vi "Write DataDVR.vi"(8 "error in (no error)":errorcluster, 10 "DataDVR":refnum<data-value>, 11 "gController in":refnum<class "gController.lvclass">) -> (0 "error out":errorcluster, 3 "gController out":refnum<class "gController.lvclass">)   [LabVIEW 2016, in "Controller.lvlib" / "gController.lvclass"]
uses:
  gController.lvclass
  Data/gData/gData.lvclass
  gController.lvclass/gController.ctl
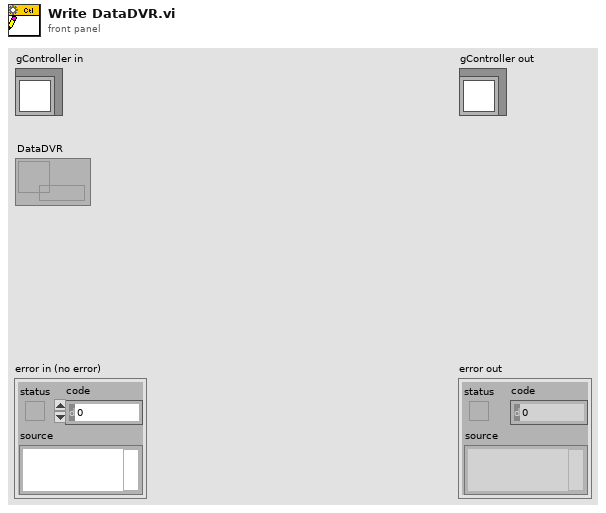
[diagram p1: front panel]
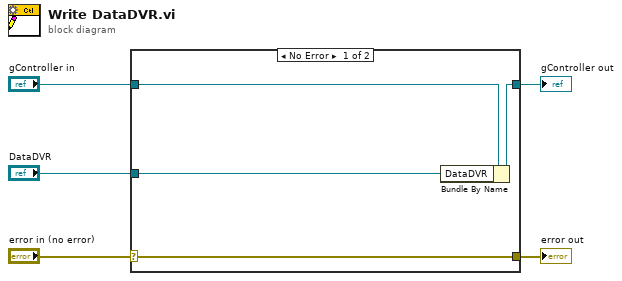
[diagram p0: block diagram]
diagram:
  n1 = case shown="No Error" "error in (no error)" {
    selector: "error in (no error)" -> [w9 w10]
    tunnel: [w9 w10] -> w4
    tunnel: [w7 w11] -> w2
    tunnel: "gController in" -> [w8 w11]
    tunnel: "DataDVR" -> [w6 _]
    frame No Error {
      n2 = Bundle By Name(cluster=w8, "DataDVR"=w6) -> (w7:refnum<class "gController.lvclass">)
    }
    frame Error {
    }
  }
  "error out" <- w4
  "gController out" <- w2
